vi "Example1.vi"() -> ()   [LabVIEW 2019]
panel:
  in  "X End":dbl
  in  "X Start":dbl
  in  "Number of Points":dbl
  out "XY Graph":cluster{dbl[], dbl[]}(graph)
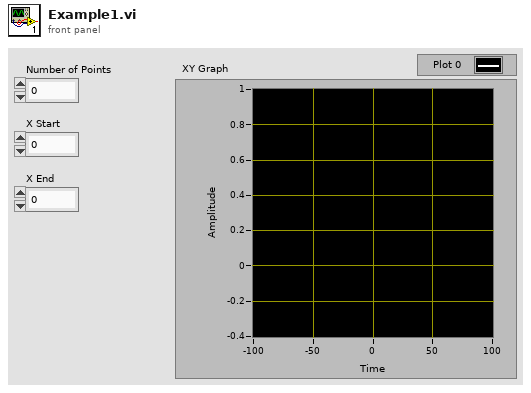
[diagram p1: front panel]
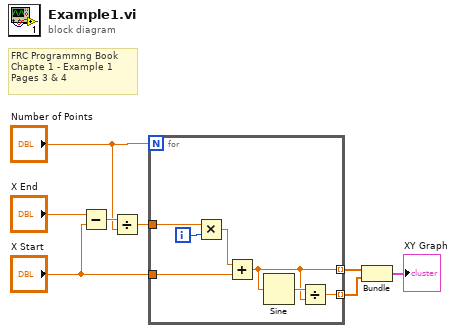
[diagram p0: block diagram]
diagram:
  # "FRC Programmng Book\nChapte 1 - Example 1\nPages 3 & 4"
  n1 = Subtract(x="X End", y="X Start") -> (x-y=w7:dbl)
  n2 = Divide(x=w7, y="Number of Points") -> (x/y=w4:dbl)
  n3 = for {
    N: "Number of Points" -> [_]
    tunnel: "X Start" -> [w12]
    tunnel: w4 -> [w15]
    tunnel: [w10] -> w3 mode=indexing
    tunnel: [w9] -> w2 mode=indexing
    i -> [w14]
    n4 = Multiply(x=w15, y=w14) -> (x*y=w13:dbl)
    n5 = Add(x=w13, y=w12) -> (x+y=w10:dbl)
    n6 = Sine(x=w10) -> (sin(x)=w11:dbl)
    n7 = Divide(x=w11, y=w10) -> (x/y=w9:dbl)
  }
  n8 = Bundle(w3, w2) -> (→"XY Graph":cluster{dbl[], dbl[]})  [unwired: 1 in]
